vi "Begin.vi"(8 "error in":errorcluster) -> (0 "error out":errorcluster)   [LabVIEW 2017]
doc: "Called before other user functions, this VI is expected to open initial I/O refnums, load in file data, and do all program initialization. Notice that the <B>error out</B> terminal is simply used for data flow. Wiring it to other structures or subVIs ensures that this VI runs first."
uses:
  <vilib>/Rock Robotics/WPI/DriverStation/WPI_DriverStationRobotMode2.ctl
  <vilib>/Rock Robotics/WPI/Joystick/WPI_JoystickDeviceEnum.ctl
  <vilib>/Rock Robotics/SystemInterfaces/DIO/FPGA_DIOPWMChannel.ctl
  <vilib>/Rock Robotics/WPI/SafetyOutput/WPI_SafetyOutputConfigMenu.ctl
  <vilib>/Rock Robotics/SystemInterfaces/spilib/spi_bus.ctl
  <vilib>/Rock Robotics/WPI/ThirdParty/Phoenix-LabVIEW/Motor Controller/Controls/CTRE_Phoenix_MotorControl_FeedbackDevice.ctl
  Robot Global Data.vi
  <vilib>/Rock Robotics/Network Tables/NT Write String Array.vi
  <vilib>/Rock Robotics/WPI/MotorControl/WPI_MotorControlOpen SPARK.vi
  <vilib>/Rock Robotics/WPI/RobotDrive/WPI_RobotDriveOpen2MotorWithVictorSP.vi
  <vilib>/Rock Robotics/WPI/RobotDrive/WPI_RobotDriveOpen4MotorWithExistingMotors.vi
  <vilib>/Rock Robotics/SystemInterfaces/AI/FPGA_AIChannel.ctl
  <vilib>/Rock Robotics/WPI/Ultrasonic/WPI_SonarSRF04DigitalRefNum Registry Set.vi
  <vilib>/Rock Robotics/WPI/Ultrasonic/WPI_SonarSRF04DigitalOpen.vi
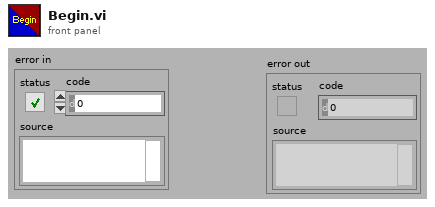
[diagram p1: front panel]
types:
  T1 = typedef "CTRE_Phoenix_MotorControl_FeedbackDevice.ctl" = i8
  T2 = typedef "WPI_SafetyOutputConfigMenu.ctl" = enum16{"Enable", "Disable"}
  T3 = typedef "FPGA_DIOPWMChannel.ctl" = enum8{"PWM 0", "PWM 1", "PWM 2", "PWM 3", "PWM 4", "PWM 5", "PWM 6", "PWM 7", "PWM 8", "PWM 9", "PWM MXP 0", "PWM MXP 1", "PWM MXP 2", "PWM MXP 3", "PWM MXP 4", "PWM MXP 5", "PWM MXP 6", "PWM MXP 7", "PWM MXP 8", "PWM MXP 9", "Invalid"}
  T4 = typedef "spi_bus.ctl" = enum16{"SPI On-Board, CS0", "SPI On-Board, CS1", "SPI On-Board, CS2", "SPI On-Board, CS3", "SPI MXP", "Invalid"}
  T5 = typedef "WPI_JoystickDeviceEnum.ctl" = enum16{"USB 0", "USB 1", "USB 2", "USB 3", "USB 4", "USB 5"}
  T6 = typedef "WPI_DriverStationRobotMode2.ctl" = enum16{"Autonomous Disabled", "Autonomous Enabled", "Teleop Disabled", "Teleop Enabled", "Disconnected", "Finish", "Test Disabled", "Test Enabled", "Emergency Stopped"}
  T7 = typedef "FPGA_AIChannel.ctl" = enum8{"AI 0", "AI 1", "AI 2", "AI 3", "AI MXP 0", "AI MXP 1", "AI MXP 2", "AI MXP 3", "Invalid"}
  T8 = typedef "WPI_UltrasonicDeviceRef.ctl" = cluster{"DevStatus":errorcluster, "Ping Channel":T9, "Echo Channel":T9, "CntIndex":T10}
  T9 = typedef "FPGA_DIOChannel.ctl" = enum8{"DIO 0", "DIO 1", "DIO 2", "DIO 3", "DIO 4", "DIO 5", "DIO 6", "DIO 7", "DIO 8", "DIO 9", "DIO MXP 0", "DIO MXP 1", "DIO MXP 2", "DIO MXP 3", "DIO MXP 4", "DIO MXP 5", "DIO MXP 6", "DIO MXP 7", "DIO MXP 8", "DIO MXP 9", "DIO MXP 10", "DIO MXP 11", "DIO MXP 12", "DIO MXP 13", "DIO MXP 14", "DIO MXP 15", "SPI Port CS1", "SPI Port CS2", "SPI Port CS3", "SPI Port MISO", "SPI Port MOSI", "Invalid"}
  T10 = typedef "FPGA_CounterCtrSystemIndex.ctl" = enum8{"Ctr 0", "Ctr 1", "Ctr 2", "Ctr 3", "Ctr 4", "Ctr 5", "Ctr 6", "Ctr 7", "Invalid"}
  T11 = typedef "WPI_MotorControlDeviceRef.ctl" = cluster{"DeviceStatus":errorcluster, "Type":T12, "PWM":cluster{"PWM Channel":T3, "DeadBand":T13}, "CAN":cluster{"Device Number":u8, "SetOutput VI Ref":variant, "GetOutput VI Ref":variant, "Enable VI Ref":variant, "Disable VI Ref":variant, "Data":variant}, "Invert":bool, "DIO PWM":cluster{"PWM \"Enable\" Channel":T3, "DIOChannel":T9, "PWM Rate":dbl}}
  T12 = typedef "WPI_MotorControlType.ctl" = enum16{"PWM", "CAN", "DIO PWM"}
  T13 = typedef "WPI_PWMDeadband.ctl" = cluster{"Name":string, "maxPositivePwm":i32, "minPositivePwm":i32, "centerPwm":i32, "maxNegativePwm":i32, "minNegativePwm":i32, "angularRange":u16}
  T14 = typedef "WPI_JoystickDevRef.ctl" = cluster{"Device":T5}
  T15 = typedef "WPI_GyroDevRef.ctl" = cluster{"DevStatus":errorcluster, "Analog Channel":T7, "Gain (VoltsPerDegree/Second)":dbl, "Gyro Type":enum16{"Analog", "XRS450"}, "Handle":i32, "SPI Bus":T4, "Device Found":bool, "Sample Rate":dbl, "Calibrate On Open":bool, "Offset":dbl}
  T16 = typedef "WPI_RobotDriveDevRef.ctl" = cluster{"DevStatus":errorcluster, "Motors[]":T11[], "Square Inputs":bool, "Max Output":dbl}
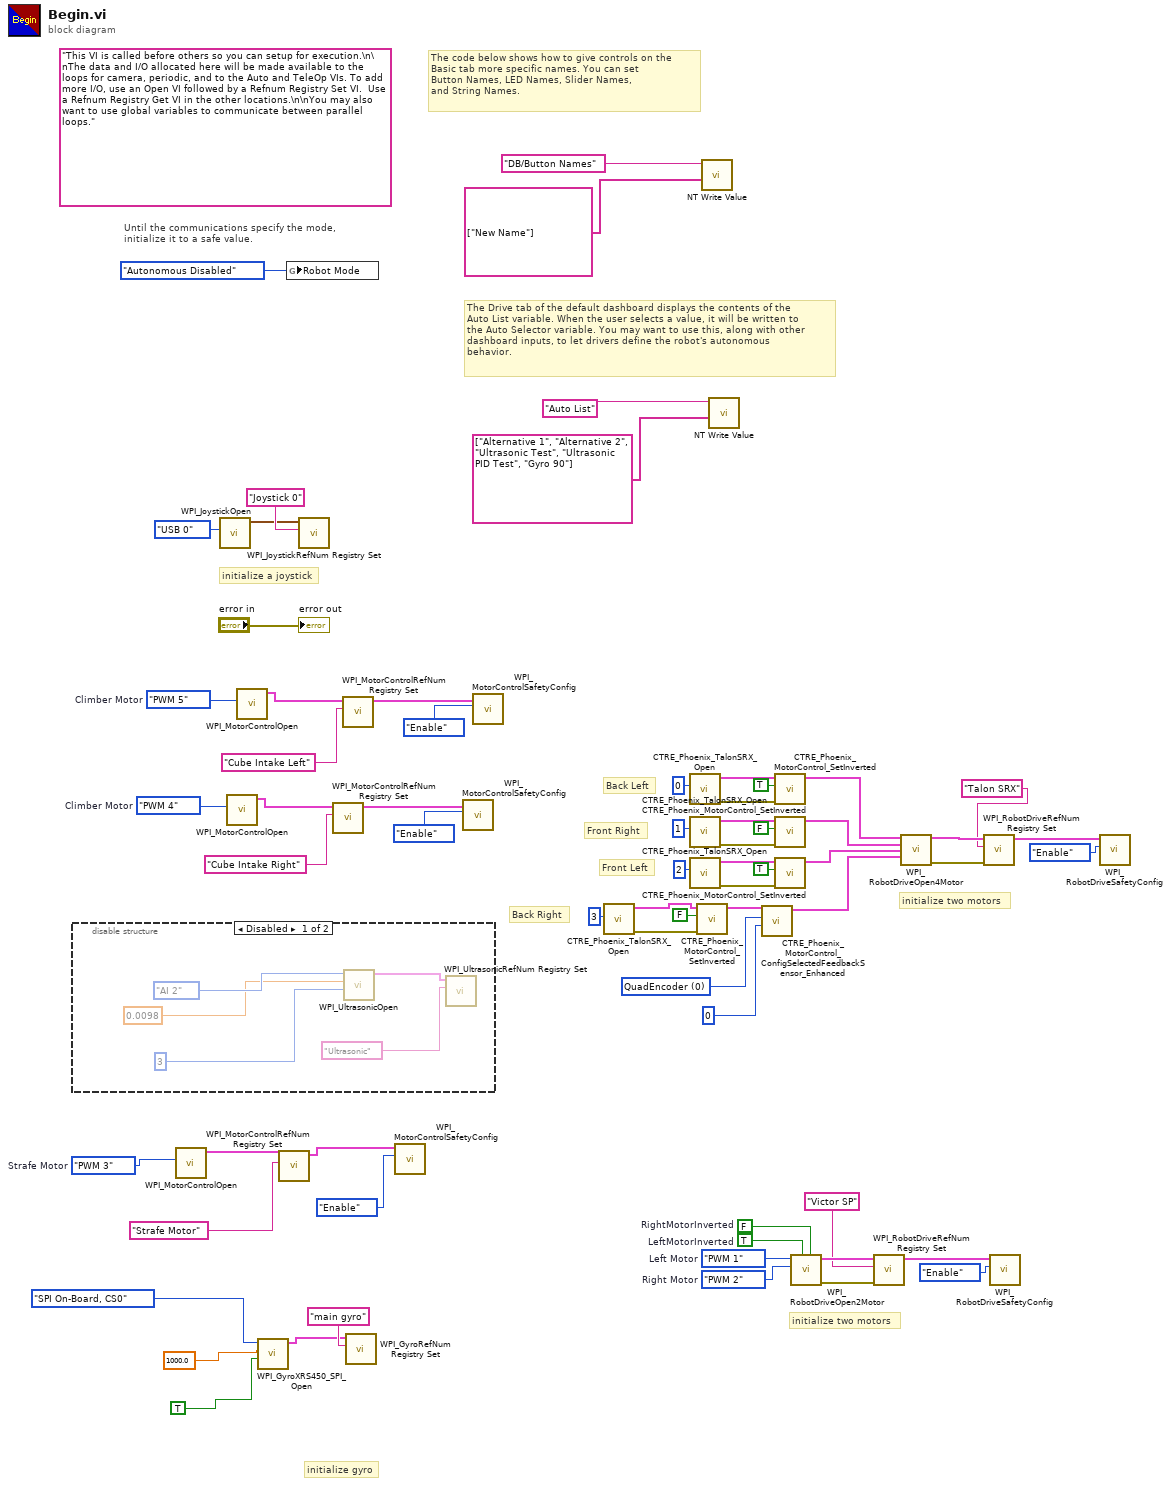
[diagram p0: block diagram]
diagram:
  w6 = T1 0 items=["None"=-1, "QuadEncoder"=0, "Analog"=2, "Tachometer"=4, "Pulse Width Encoded Position"=8, "Sensor Sum (S0 + S1)"=9, "Sensor Difference (D0 - D1)"=10, "Remote Source 0"=11, "Remote Source 1"=12, "Software Emulated"=15] ("Feedback Device")
  w10 = FPGA_DIOPWMChannel."PWM 2"  # Right Motor
  w9 = FPGA_DIOPWMChannel."PWM 1"  # Left Motor
  w11 = TRUE  # LeftMotorInverted
  w12 = FALSE  # RightMotorInverted
  w47 = FPGA_DIOPWMChannel."PWM 3"  # Strafe Motor
  w49 = FPGA_DIOPWMChannel."PWM 4"  # Climber Motor
  w56 = FPGA_DIOPWMChannel."PWM 5"  # Climber Motor
  (unwired) "This VI is called before others so you can setup for execution.\n\nThe data and I/O allocated here will be made available to the loops for camera, periodic, and to the Auto and TeleOp VIs. To add more I/O, use an Open VI followed by a Refnum Registry Set VI.  Use a Refnum Registry Get VI in the other locations.\n\nYou may also want to use global variables to communicate between parallel loops."
  # "initialize two motors"
  # "Back Right"
  # "Front Left"
  # "Front Right"
  # "Back Left"
  # "initialize two motors"
  # "initialize gyro"
  # "The Drive tab of the default dashboard displays the contents of the\nAuto List variable. When the user selects a value, it will be written to\nthe Auto Selector variable. You may want to use this, along with other\ndashboard inputs, to let drivers define the robot's autonomous\nbehavior."
  # "The code below shows how to give controls on the\nBasic tab more specific names. You can set\nButton Names, LED Names, Slider Names,\nand String Names."
  # "initialize a joystick"
  # "Until the communications specify the mode,\ninitialize it to a safe value."
  n1 = disable-structure shown="Disabled" {
    frame Disabled {
      n2 = call-poly <vilib>:"WPI_UltrasonicOpen.vi"("Echo DIO Channel"=3, 10:0.0098, "Ping DIO Channel"=FPGA_AIChannel."AI 2" ("Channel")) -> ("SonarSRF04DevRef"=w68:T8)  [unwired: 7 in, 1 out]
      n3 = call-poly <vilib>:"WPI_UltrasonicRefNum Registry Set.vi"("refnum name"="Ultrasonic", "SonarSRF04DevRef"=w68) -> ()  [unwired: 8 in, 2 out]
    }
    frame Enabled {
    }
  }
  n4 = call-poly <vilib>:"WPI_MotorControlOpen.vi"("PWM Channel"=w47) -> ("MotorControlDeviceRef"=w46:T11)  [unwired: 9 in, 1 out]
  n5 = call <vilib>:"WPI_JoystickOpen.vi"("JoystickDevice"=WPI_JoystickDeviceEnum."USB 0") -> ("JoystickDevRef"=w64:T14)  [unwired: 10 in]
  n6 = call-poly <vilib>:"WPI_MotorControlOpen.vi"("PWM Channel"=w49) -> ("MotorControlDeviceRef"=w48:T11)  [unwired: 9 in, 1 out]
  n7 = call-poly <vilib>:"WPI_MotorControlOpen.vi"("PWM Channel"=w56) -> ("MotorControlDeviceRef"=w57:T11)  [unwired: 9 in, 1 out]
  n8 = call <vilib>:"WPI_GyroXRS450_SPI_Open.vi"("Calibrate On Open"=TRUE, "Sample Rate (Hz)"=1000.0, "SPI Bus"=spi_bus."SPI On-Board, CS0") -> ("GyroDevRef"=w38:T15)  [unwired: 6 in, 2 out]
  n9 = call <vilib>:"WPI_MotorControlRefNum Registry Set.vi"("refnum name"="Strafe Motor", "MotorControlDevRef"=w46) -> ("MotorControlDevRef"=w44:T11)  [unwired: 8 in, 1 out]
  n10 = global write "Robot Global Data.vi" "Robot Mode"(WPI_DriverStationRobotMode2."Autonomous Disabled" ("Robot Mode")) -> ()
  n11 = call <vilib>:"WPI_JoystickRefNum Registry Set.vi"("refnum name"="Joystick 0", "JoystickDevRef"=w64) -> ()  [unwired: 8 in, 2 out]
  n12 = call <vilib>:"WPI_MotorControlRefNum Registry Set.vi"("refnum name"="Cube Intake Right", "MotorControlDevRef"=w48) -> ("MotorControlDevRef"=w50:T11)  [unwired: 8 in, 1 out]
  n13 = call <vilib>:"WPI_MotorControlRefNum Registry Set.vi"("refnum name"="Cube Intake Left", "MotorControlDevRef"=w57) -> ("MotorControlDevRef"=w55:T11)  [unwired: 8 in, 1 out]
  n14 = call <vilib>:"WPI_GyroRefNum Registry Set.vi"("refnum name"="main gyro", "GyroDevRef"=w38) -> ()  [unwired: 8 in, 2 out]
  n15 = call <vilib>:"WPI_MotorControlSafetyConfig.vi"("mode"=WPI_SafetyOutputConfigMenu."Enable", "MotorControlDevRef"=w44) -> ()  [unwired: 8 in, 2 out]
  n16 = call <vilib>:"WPI_MotorControlSafetyConfig.vi"("mode"=WPI_SafetyOutputConfigMenu."Enable", "MotorControlDevRef"=w50) -> ()  [unwired: 8 in, 2 out]
  n17 = call <vilib>:"WPI_MotorControlSafetyConfig.vi"("mode"=WPI_SafetyOutputConfigMenu."Enable", "MotorControlDevRef"=w55) -> ()  [unwired: 8 in, 2 out]
  n18 = call <vilib>:"CTRE_Phoenix_TalonSRX_Open.vi"("Device Number"=u8 3) -> ("error out"=w3:errorcluster, "CAN Talon SRX Ref"=w4:T11)  [unwired: 9 in]
  n19 = call <vilib>:"CTRE_Phoenix_TalonSRX_Open.vi"("Device Number"=u8 0) -> ("error out"=w37:errorcluster, "CAN Talon SRX Ref"=w36:T11)  [unwired: 9 in]
  n20 = call <vilib>:"CTRE_Phoenix_TalonSRX_Open.vi"("Device Number"=u8 1) -> ("error out"=w29:errorcluster, "CAN Talon SRX Ref"=w30:T11)  [unwired: 9 in]
  n21 = call <vilib>:"CTRE_Phoenix_TalonSRX_Open.vi"("Device Number"=u8 2) -> ("error out"=w34:errorcluster, "CAN Talon SRX Ref"=w33:T11)  [unwired: 9 in]
  n22 = call <vilib>:"CTRE_Phoenix_MotorControl_SetInverted.vi"("error in (no error)"=w3, "Invert?"=FALSE, "PhoenixMotorControlDevRef"=w4) -> ("PhoenixMotorControlDevRef"=w2:T11)  [unwired: 7 in, 1 out]
  n23 = call-poly <vilib>:"NT Write Value.vi"("String Array"=string[] ["New Name"], "Name"="DB/Button Names") -> ()  [unwired: 9 in, 1 out]
  n24 = call-poly <vilib>:"NT Write Value.vi"("String Array"=string[] ["Alternative 1", "Alternative 2", "Ultrasonic Test", "Ultrasonic PID Test", "Gyro 90"], "Name"="Auto List") -> ()  [unwired: 9 in, 1 out]
  n25 = call <vilib>:"CTRE_Phoenix_MotorControl_ConfigSelectedFeedbackSensor_Enhanced.vi"("pidLoopIdx"=u8 0 ("Device Number"), "Feedback Device"=w6, "PhoenixMotorControlDevRef"=w2) -> ("PhoenixMotorControlDevRef"=w1:T11)  [unwired: 7 in, 1 out]
  n26 = call <vilib>:"CTRE_Phoenix_MotorControl_SetInverted.vi"("error in (no error)"=w37, "Invert?"=TRUE, "PhoenixMotorControlDevRef"=w36) -> ("PhoenixMotorControlDevRef"=w35:T11)  [unwired: 7 in, 1 out]
  n27 = call <vilib>:"CTRE_Phoenix_MotorControl_SetInverted.vi"("error in (no error)"=w29, "Invert?"=FALSE, "PhoenixMotorControlDevRef"=w30) -> ("PhoenixMotorControlDevRef"=w31:T11)  [unwired: 7 in, 1 out]
  n28 = call <vilib>:"CTRE_Phoenix_MotorControl_SetInverted.vi"("error in (no error)"=w34, "Invert?"=TRUE, "PhoenixMotorControlDevRef"=w33) -> ("PhoenixMotorControlDevRef"=w32:T11)  [unwired: 7 in, 1 out]
  n29 = call-poly <vilib>:"WPI_RobotDriveOpen2Motor.vi"("Right Motor Inverted"=w12, "Left Motor Inverted"=w11, "Right Motor"=w10, "Left Motor"=w9) -> ("error out"=w15:errorcluster, "RobotDriveDevRef"=w16:T16)  [unwired: 1 in, 5 out]
  n30 = call <vilib>:"WPI_RobotDriveRefNum Registry Set.vi"("error in (no error)"=w15, "refnum name"="Victor SP", "RobotDriveDevRef"=w16) -> ("RobotDriveDevRef"=w14:T16)  [unwired: 1 in, 7 out]
  n31 = call-poly <vilib>:"WPI_RobotDriveOpen4Motor.vi"("Rear Left Motor Dev Ref"=w35, "Rear Right Motor Dev Ref"=w31, "Front Left Motor Dev Ref"=w32, "Front Right Motor Dev Ref"=w1) -> ("RobotDriveDevRef"=w26:T16, "error out"=w27:errorcluster)  [unwired: 10 in]
  n32 = call <vilib>:"WPI_RobotDriveRefNum Registry Set.vi"("error in (no error)"=w27, "refnum name"="Talon SRX", "RobotDriveDevRef"=w26) -> ("RobotDriveDevRef"=w28:T16)  [unwired: 1 in, 7 out]
  n33 = call <vilib>:"WPI_RobotDriveSafetyConfig.vi"("mode"=WPI_SafetyOutputConfigMenu."Enable", "RobotDriveDevRef"=w14) -> ()  [unwired: 8 in, 2 out]
  n34 = call <vilib>:"WPI_RobotDriveSafetyConfig.vi"("mode"=WPI_SafetyOutputConfigMenu."Enable", "RobotDriveDevRef"=w28) -> ()  [unwired: 8 in, 2 out]
  "error out" <- "error in"
